vi "StartZTAlignmentInitAbsMove.vi"(8 "error in (no error)":errorcluster, 9 "Z, mm, T deg":dbl[](array[numeric]), 11 "VXMMotionManager in":refnum<class "VXMMotionManager.lvclass">) -> (0 "error out":errorcluster, 3 "VXMMotionManager out":refnum<class "VXMMotionManager.lvclass">)   [LabVIEW 2018, in "VXMMotionManager.lvclass"]
doc: "Load up X position and Y position and go to the start and move case.\n\n**CAUTION** This absolute move does not move the probe up and out of the way.\n It moves in X and Y only in order s[eed up the alignment. \n Also, the alignment should be performed at a high Z position."
uses:
  VXMMotionManager.lvclass
  MoveAllAbsoluteStates.ctl
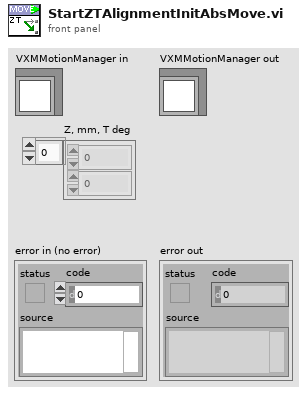
[diagram p1: front panel]
types:
  T1 = typedef "VXMMotionManager.lvclass/MoveAllAbsoluteStates.ctl" = enum16{"start next move", "wait motion end"}
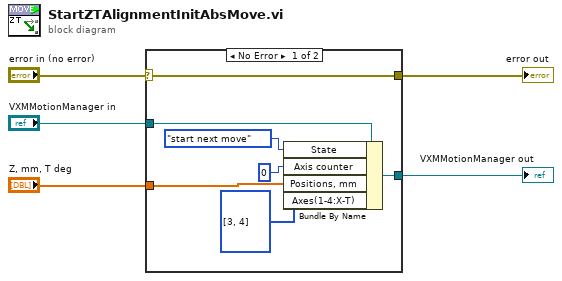
[diagram p0: block diagram]
diagram:
  n1 = case shown="No Error" "error in (no error)" {
    selector: "error in (no error)" -> [w12 w14]
    tunnel: [w12 w14] -> w2
    tunnel: [w10 w13] -> w3
    tunnel: "VXMMotionManager in" -> [w8 w13]
    tunnel: "Z, mm, T deg" -> [w7 _]
    frame No Error {
      n2 = Bundle By Name(cluster=w8, "State"=MoveAllAbsoluteStates."start next move", "Axis counter"=0 ("Axis (0-3)"), "Positions, mm"=w7, "Axes(1-4:X-T)"=i32[] [3, 4] ("Axes(1-4:X-R)")) -> (w10:refnum<class "VXMMotionManager.lvclass">)
    }
    frame Error {
    }
  }
  "error out" <- w2
  "VXMMotionManager out" <- w3
